vi "_close_.vi"(8 "error in":errorcluster, 11 "Coarse Approach.lvclass":refnum<class "Coarse Approach.lvclass">) -> (0 "error out":errorcluster)   [LabVIEW 2020, in "Coarse Approach.lvclass"]
uses:
  Coarse Approach.lvclass
  Coarse Approach.lvclass/Coarse Approach.ctl
  Lock-In Amplifier/Lock-In Amplifier.lvclass
  Function Generator/Function Generator.lvclass
  Newport Model 8742/New Focus Model 8742.lvclass
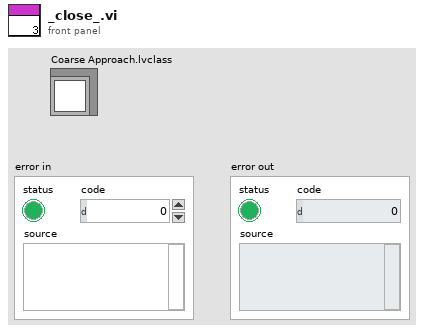
[diagram p1: front panel]
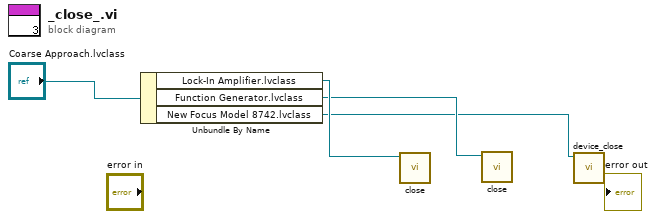
[diagram p0: block diagram]
diagram:
  n1 = Unbundle By Name("Coarse Approach.lvclass") -> ("Lock-In Amplifier.lvclass"=w3:refnum<class "Lock-In Amplifier.lvclass">, "Function Generator.lvclass"=w2:refnum<class "Function Generator.lvclass">, "New Focus Model 8742.lvclass"=w1:refnum<class "New Focus Model 8742.lvclass">)
  n2 = call-dynamic "close.vi"("Instrument in"=w3) -> ()  [unwired: 10 in, 1 out]
  n3 = call-dynamic "close.vi"("Function Generator in"=w2) -> ()  [unwired: 10 in, 1 out]
  n4 = call "device_close.vi"("New Focus Model 8742.lvclass"=w1) -> ()  [unwired: 10 in, 1 out]
